vi "Show Disconnected Msg.vi"(8 "error in (no error)":errorcluster, 11 "CS++GoBangClient in":refnum<class "CS++GoBangClient.lvclass">) -> (0 "error out":errorcluster, 3 "CS++GoBangClient out":refnum<class "CS++GoBangClient.lvclass">)   [LabVIEW 2014, in "GoBang.lvlib" / "CS++GoBangClient.lvclass"]
uses:
  CS++GoBangClient.lvclass
  CS++GoBangServer Messages/Reset Board Msg/Reset Board Msg.lvclass
  CS++GoBangClient.lvclass/CS++GoBangClient.ctl
  <vilib>/NI/Actors/Linked Network Actor/Linked Network Actor Messages/Transmit Network Message Msg/Transmit Network Message Msg.lvclass
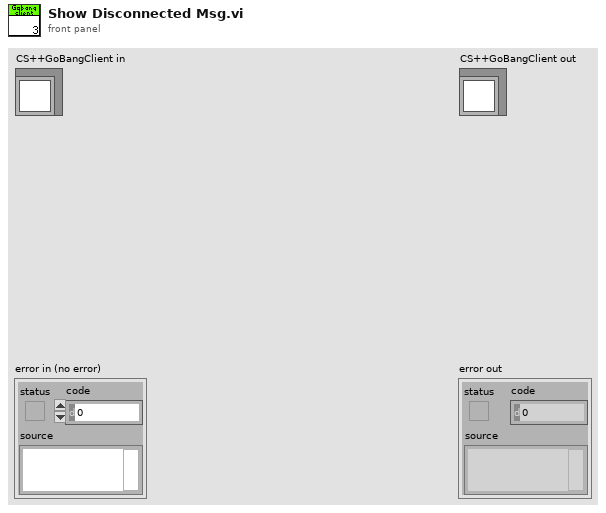
[diagram p1: front panel]
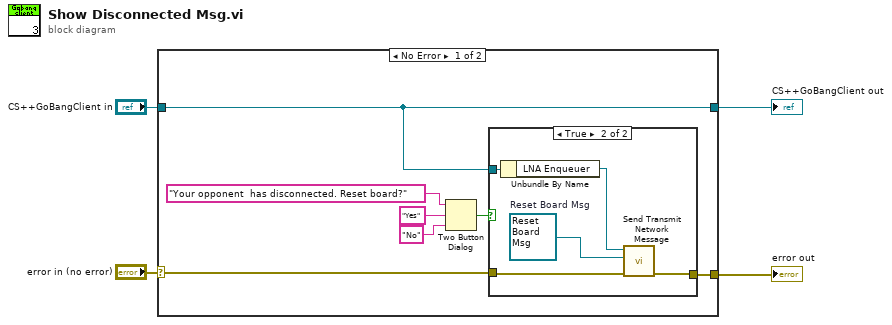
[diagram p0: block diagram]
diagram:
  n1 = case shown="No Error" "error in (no error)" {
    selector: "error in (no error)" -> [w5 w19]
    tunnel: [w6 w19] -> w3
    tunnel: [w7 w18] -> w1
    tunnel: "CS++GoBangClient in" -> [w7 w18]
    frame No Error {
      n2 = Two Button Dialog(message="Your opponent  has disconnected. Reset board?" ("string"), 1:"No" ("F button name (\"Cancel\")"), 2:"Yes" ("T button name (\"OK\")")) -> (T button?=w11:bool)
      n3 = case shown="True" w11 {
        tunnel: w7 -> [_ w17]
        tunnel: [w12 w14] -> w6
        tunnel: w5 -> [w12 w13]
        frame False {
        }
        frame True {
          w15 = refnum<class "Reset Board Msg.lvclass"> refnum  # Reset Board Msg
          n4 = Unbundle By Name(w17) -> ("LNA Enqueuer"=w16:refnum<class "Message Enqueuer.lvclass">)
          n5 = call <vilib>:"Send Transmit Network Message.vi"("error in (no error)"=w13, "Message"=w15, "Message Enqueuer"=w16) -> ("error out"=w14:errorcluster)  [unwired: 7 in, 1 out]
        }
      }
    }
    frame Error {
    }
  }
  "error out" <- w3
  "CS++GoBangClient out" <- w1
